vi "Set MFC Gase.vi"(8 "Fehler (Eingang, kein Fehler)":errorcluster, 11 "HovaCAL MFC Gase Cluster":cluster{"MFC Gasauswahl":u16}[](array[cluster]) caption="MFC Gase" {"MFC Gasauswahl" items=["Air"]}) -> (0 "Fehler (Ausgang)":errorcluster, 3 "mfc Gasnamen out":string[](array[string]))   [LabVIEW 2020, in "Linearisierung v2.lvlib" / "Gasteiler.lvlib" / "HovaCAL_Interface.lvlib" / "Kommunikation.lvlib"]
uses:
  Kommunikation.lvlib
  Aktion_FGV_HovaCAL_Interface_Gasliste.ctl
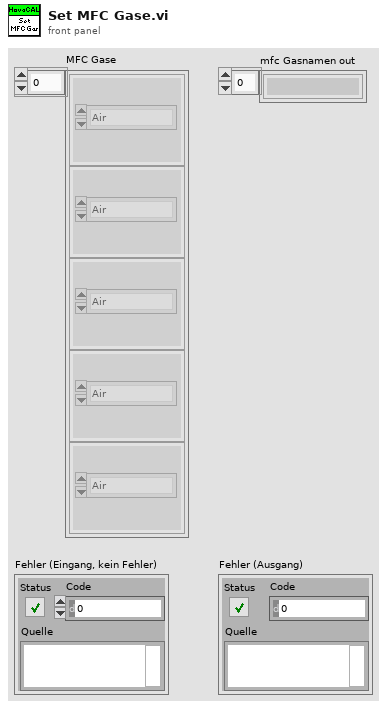
[diagram p1: front panel]
types:
  T1 = typedef "Linearisierung v2.lvlib/Gasteiler.lvlib/HovaCAL_Interface.lvlib/Kommunikation.lvlib/Aktion_FGV_HovaCAL_Interface_Gasliste.ctl" = enum16{"lesen", "setzen", "erstellen"}
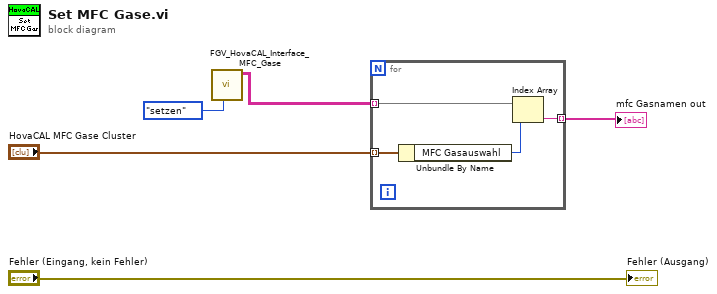
[diagram p0: block diagram]
diagram:
  n1 = call "FGV_HovaCAL_Interface_MFC_Gase.vi"("Aktion"=Aktion_FGV_HovaCAL_Interface_Gasliste."setzen") -> ("mfc Gaslisten out"=w3:string[][])  [unwired: 8 in, 2 out]
  n2 = for {
    tunnel: "HovaCAL MFC Gase Cluster" -> [w9] mode=indexing
    tunnel: w3 -> [w7] mode=indexing
    tunnel: [w6] -> w2 mode=indexing
    n3 = Unbundle By Name(w9) -> ("MFC Gasauswahl"=w8:u16)
    n4 = Index Array(array=w7, index=w8) -> (element=w6:string)
  }
  "mfc Gasnamen out" <- w2
  "Fehler (Ausgang)" <- "Fehler (Eingang, kein Fehler)"
